vi "hmi_initialize.vi"(7 "hmi_references":T1, 8 "error in (no error)":errorcluster) -> (0 "error out":errorcluster)   [LabVIEW 2015, in "lv-build-interface.lvlib"]
uses:
  lv-build-interface.lvlib
  _controls/hmi_references.ctl
  _controls/navigation.ctl
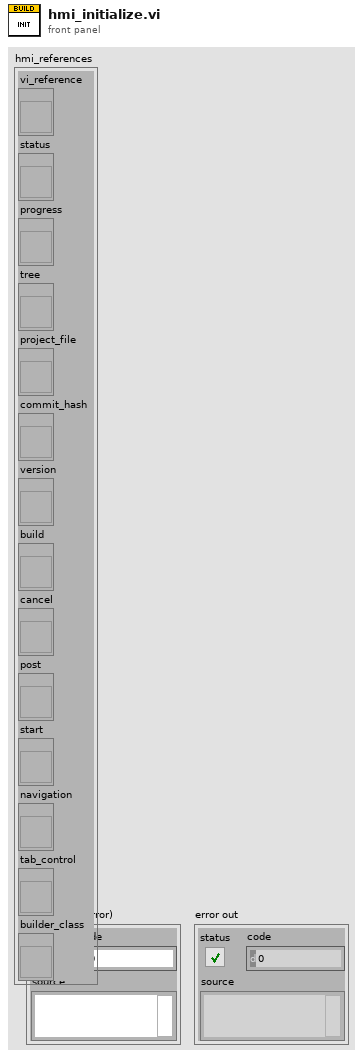
[diagram p1: front panel]
types:
  T1 = typedef "lv-build-interface.lvlib/hmi_references.ctl" = cluster{"vi_reference":refnum<vi>, "status":refnum<vi>, "progress":refnum<vi>, "tree":refnum<vi>, "project_file":refnum<vi>, "commit_hash":refnum<vi>, "version":refnum<vi>, "build":refnum<vi>, "cancel":refnum<vi>, "post":refnum<vi>, "start":refnum<vi>, "navigation":refnum<vi>, "tab_control":refnum<vi>, "builder_class":refnum<vi>}
  T2 = typedef "lv-build-interface.lvlib/navigation.ctl" = enum32{"tool", "build"}
  T3 = enum8{"Enabled", "Disabled", "Disabled and Grayed Out"}
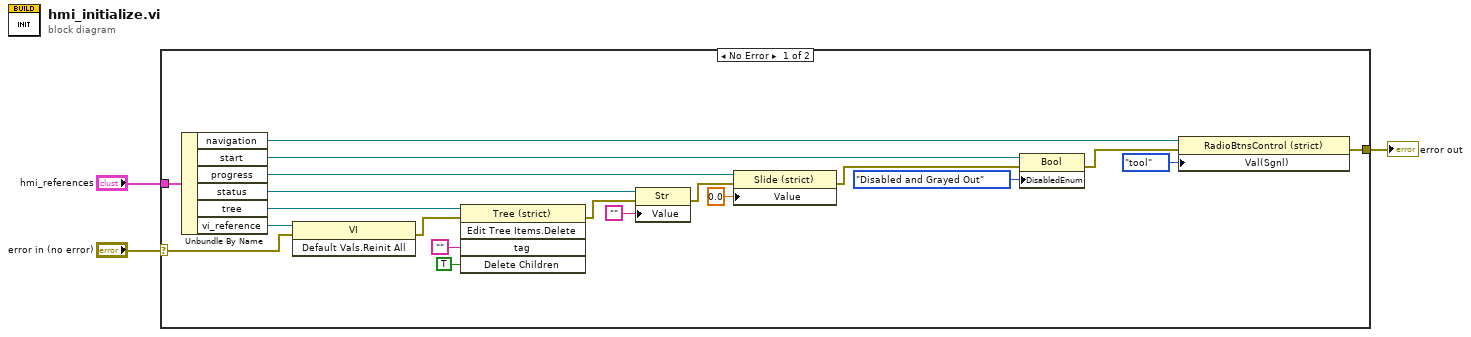
[diagram p0: block diagram]
diagram:
  n1 = case shown="No Error" "error in (no error)" {
    selector: "error in (no error)" -> [w8 w24]
    tunnel: [w6 w24] -> w2
    tunnel: "hmi_references" -> [w23 _]
    frame No Error {
      n2 = Unbundle By Name(w23) -> ("navigation"=w7:refnum<vi>, "start"=w12:refnum<vi>, "progress"=w18:refnum<vi>, "status"=w19:refnum<vi>, "tree"=w22:refnum<vi>, "vi_reference"=w9:refnum<vi>)
      n3 = invoke class="VI" method="Default Vals.Reinit All"(reference=w9, error in=w8) -> (error out=w13:errorcluster)  [unwired: 1 in, 2 out]
      n4 = invoke class="Tree (strict)" method="Edit Tree Items.Delete"(reference=w22, error in=w13, "tag"="", "Delete Children"=TRUE ("Delete Children?")) -> (error out=w17:errorcluster)  [unwired: 1 in, 4 out]
      n5 = property class="Str"(reference=w19, error in=w17, "Value"="") -> (error out=w16:errorcluster)  [unwired: 1 out]
      n6 = property class="Slide (strict)"(reference=w18, error in=w16, "Value"=0.0) -> (error out=w11:errorcluster)  [unwired: 1 out]
      n7 = property class="Bool"(reference=w12, error in=w11, "DisabledEnum"=T3."Disabled and Grayed Out" ("Disabled")) -> (error out=w4:errorcluster)  [unwired: 1 out]
      n8 = property class="RadioBtnsControl (strict)"(reference=w7, error in=w4, "Val(Sgnl)"=navigation."tool" ("Value (Signaling)")) -> (error out=w6:errorcluster)  [unwired: 1 out]
    }
    frame Error {
    }
  }
  "error out" <- w2
